vi "ColourCheckTesting.vi"() -> ()   [LabVIEW 2022 SP3]
uses:
  Global Red.vi
  Global Green.vi
  Global Blue.vi
  final ma final ma/Reading Blue.vi
  final ma final ma/Reading Red.vi
  final ma final ma/Reading Green.vi
panel:
  out "String 3":string="blue"
  out "String 2":string="green"
  out "String":string="red"
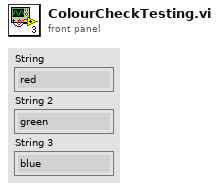
[diagram p1: front panel]
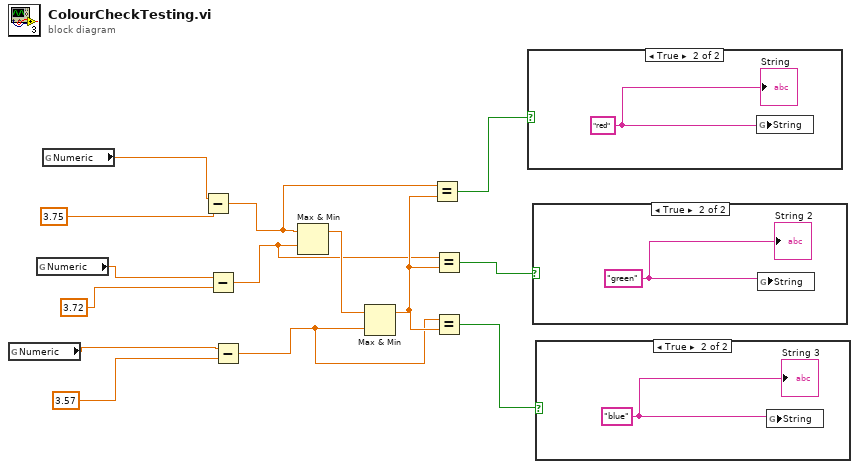
[diagram p0: block diagram]
diagram:
  n1 = global read "Reading Blue.vi" "Numeric"() -> (w1:dbl)
  n2 = global read "Reading Green.vi" "Numeric"() -> (w2:dbl)
  n3 = global read "Reading Red.vi" "Numeric"() -> (w3:dbl)
  n4 = Subtract(x=w3, y=3.75) -> (x-y=w12:dbl)
  n5 = Subtract(x=w2, y=3.72) -> (x-y=w11:dbl)
  n6 = Subtract(x=w1, y=3.57) -> (x-y=w10:dbl)
  n7 = Max & Min(x=w12, y=w11) -> (max(x,y)=w14:dbl)  [unwired: 1 out]
  n8 = Max & Min(x=w14, y=w10) -> (max(x,y)=w13:dbl)  [unwired: 1 out]
  n9 = Equal?(x=w12, y=w13) -> (x = y?=w9:bool)
  n10 = Equal?(x=w11, y=w13) -> (x = y?=w8:bool)
  n11 = Equal?(x=w10, y=w13) -> (x = y?=w7:bool)
  n12 = case shown="True" w9 {
    frame False {
    }
    frame True {
      w15 = "red"
      n13 = global write "Global Red.vi" "String"(w15) -> ()
      "String" <- w15
    }
  }
  n14 = case shown="True" w8 {
    frame False {
    }
    frame True {
      w16 = "green"
      n15 = global write "Global Green.vi" "String"(w16) -> ()
      "String 2" <- w16
    }
  }
  n16 = case shown="True" w7 {
    frame False {
    }
    frame True {
      w17 = "blue"
      n17 = global write "Global Blue.vi" "String"(w17) -> ()
      "String 3" <- w17
    }
  }
